vi "mod_frequency.vi"(7 "LVWSR":refnum<class "Web Request.lvclass">, 10 "fmod":u32, 11 "cell":u8) -> ()   [LabVIEW 2016]
uses:
  <vilib>/wsapi/Web Request.lvclass
  Controller/Messages/Forward Command/Forward Command MSG.lvclass
  C:/Program Files (x86)/National Instruments/LabVIEW 2016/vi.lib/ActorFramework/Message/Message.lvclass
  PAS/Commands/Change Laser Frequency Cmd/Change Laser Frequency CMD.lvclass
  C:/Program Files (x86)/National Instruments/LabVIEW 2016/vi.lib/MSR Consulting, LLC/General Reuse/Command/Command.lvclass
  PAS/Commands/Change Laser Frequency Cmd/Change Laser Frequency CMD.lvclass/Change Laser Frequency CMD.ctl
  Controller/Messages/Forward Command/Forward Command MSG.lvclass/Forward Command MSG.ctl
  <vilib>/ActorFramework/Message Enqueuer/Message Enqueuer.lvclass/Message Enqueuer.ctl
  PAS/Commands/Change Laser Frequency Cmd/Write Cell.vi
  PAS/Commands/Change Laser Frequency Cmd/Write f.vi
  Controller/Messages/Forward Command/Write id.vi
  Controller/Messages/Forward Command/Write CMD.vi
  <vilib>/ActorFramework/Message Priority Queue/Priority Enqueue.vi
  Controller/gController.lvclass
  <vilib>/ActorFramework/Message Enqueuer/Message Enqueuer.lvclass
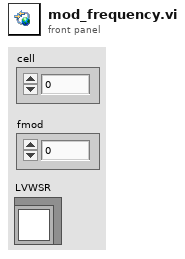
[diagram p1: front panel]
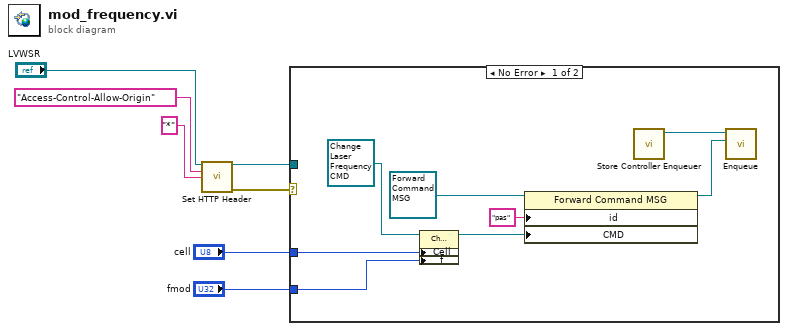
[diagram p0: block diagram]
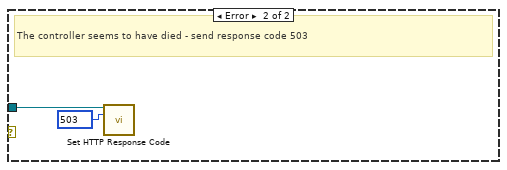
[diagram p2: hidden frame]
diagram:
  n1 = call <vilib>:"Set HTTP Header.vi"("LabVIEW Web Service Request"="LVWSR", "header"="Access-Control-Allow-Origin", "header value"="*") -> ("LabVIEW Web Service Request out"=w3:refnum<class "Web Request.lvclass">, "error out"=w2:errorcluster)  [unwired: 11 in]
  n2 = case shown="No Error" w2 {
    tunnel: w3 -> [_ w16]
    tunnel: "cell" -> [w10 _]
    tunnel: "fmod" -> [w9 _]
    frame No Error {
      n3 = property class="Change Laser Frequency CMD"(reference=refnum<class "Change Laser Frequency CMD.lvclass"> refnum ("gPAS Library.lvlib:Change Laser Frequency CMD"), "Cell"=w10, "f"=w9) -> (reference out=w11:refnum<class "Change Laser Frequency CMD.lvclass">)  [unwired: 1 in, 1 out]
      n4 = property class="Forward Command MSG"(reference=refnum<class "Forward Command MSG.lvclass"> refnum ("Controller.lvlib:Forward Command MSG.lvclass"), "id"="pas", "CMD"=w11) -> (reference out=w13:refnum<class "Forward Command MSG.lvclass">)  [unwired: 1 in, 1 out]
      n5 = call "Store Controller Enqueuer.vi"() -> ("Controller Enqueuer Out"=w15:refnum<class "Message Enqueuer.lvclass">)  [unwired: 11 in]
      n6 = call <vilib>:"Enqueue.vi"("Message"=w13, "Message Enqueuer in"=w15) -> ()  [unwired: 8 in, 2 out]
    }
    frame Error {
      w17 = 503 items=["100"=100, "101"=101, "200"=200, "201"=201, "202"=202, "203"=203, "204"=204, "205"=205, "206"=206, "300"=300, "301"=301, "302"=302, "303"=303, "304"=304, "305"=305, "306"=306, "307"=307, "400"=400, "401"=401, "402"=402, "403"=403, "404"=404, "405"=405, "406"=406, "407"=407, "408"=408, "409"=409, "410"=410, "411"=411, "412"=412, "413"=413, "414"=414, "415"=415, "416"=416, "417"=417, "500"=500, "501"=501, "502"=502, "503"=503, "504"=504, "505"=505] ("response code (200)")
      # "The controller seems to have died - send response code 503"
      n7 = call <vilib>:"Set HTTP Response Code.vi"("LabVIEW Web Service Request"=w16, "response code (200)"=w17) -> ()  [unwired: 12 in, 2 out]
    }
  }
